vi "Cleanup.vi"(8 "error in (no error)":errorcluster, 11 "Resource in":refnum<class "Resource.lvclass">) -> (0 "error out":errorcluster)   [LabVIEW 2020, in "PicoG-Core.lvlib" / "Resource.lvclass"]
uses:
  Resource.lvclass
  Resource.lvclass/Resource.ctl
  <vilib>/IlluminatedG/lv-stream/Connection/Connection.lvclass
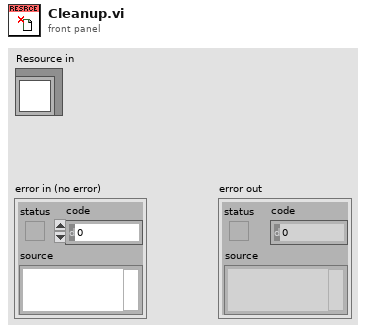
[diagram p1: front panel]
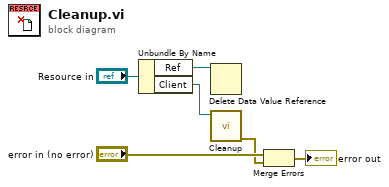
[diagram p0: block diagram]
diagram:
  n1 = Unbundle By Name("Resource in") -> ("Ref"=w4:refnum<data-value>, "Client"=w1:refnum<class "Connection.lvclass">)
  n2 = Delete Data Value Reference(data value reference=w4) -> ()  [unwired: 1 in, 2 out]
  n3 = call-dynamic "Cleanup.vi"("Connection in"=w1) -> ("error out"=w2:errorcluster)  [unwired: 10 in]
  n4 = Merge Errors("error in (no error)", w2) -> (→"error out":errorcluster)
